vi "VMUIStop.vi"(8 "error in (no error)":errorcluster, 11 "VariableManagerRef in":refnum<vi>) -> (0 "error out":errorcluster, 3 "VariableManagerRef out":refnum<vi>)   [LabVIEW 2013, in "VariableManagerAPI.lvlib"]
doc: "Stop VariableManagerUserInterface. You must call VMUIStop.vi on all started variable manager before your application exit."
uses:
  VariableManagerAPI.lvlib
  VariableManager/VariableManager.lvclass
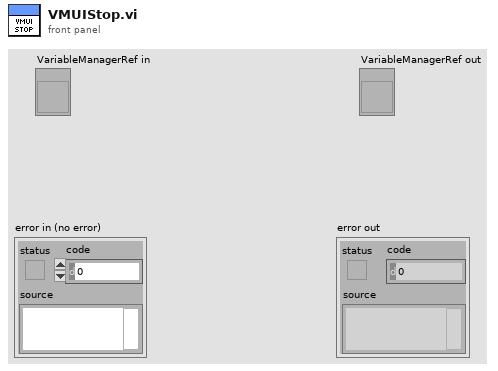
[diagram p1: front panel]
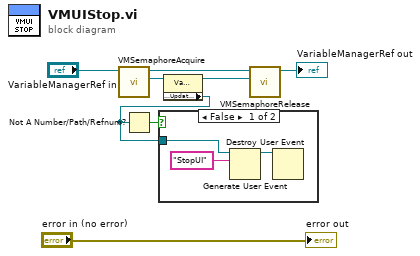
[diagram p0: block diagram]
diagram:
  n1 = call "VMSemaphoreAcquire.vi"("VariableManagerRef in"="VariableManagerRef in") -> ("VariableManager"=w4:refnum<class "VariableManager.lvclass">, "VariableManagerRef out"=w5:refnum<vi>)  [unwired: 7 in, 2 out]
  n2 = property class="VariableManager.lvclass"(reference=w4) -> (reference out=w3:refnum<class "VariableManager.lvclass">, "Accessors:UpdateEvent"=w1:refnum<user-event>)  [unwired: 1 in, 1 out]
  n3 = Not A Number/Path/Refnum?(number/path/refnum=w1) -> (NaN/Path/Refnum?=w2:bool)
  n4 = case shown="False" w2 {
    tunnel: w1 -> [w9 _]
    frame False {
      n5 = Generate User Event(user event=w9, event data cluster="StopUI") -> (user event out=w11:refnum<user-event>)  [unwired: 2 in, 1 out]
      n6 = Destroy User Event(user event=w11) -> ()  [unwired: 1 in, 1 out]
    }
    frame True {
    }
  }
  n7 = call "VMSemaphoreRelease.vi"("VariableManager"=w3, "VariableManagerRef in"=w5) -> ("VariableManagerRef out"=→"VariableManagerRef out":refnum<vi>)  [unwired: 8 in, 1 out]
  "error out" <- "error in (no error)"
